vi "GetMotorHall.vi"(7 "Hall AI":dbl[][](array[numeric]), 8 "Hall状态输入":bool[](array[boolean]), 9 "电流输入":dbl[](array[numeric]), 11 "hall in":i64[](array[numeric])) -> (0 "Hall状态输出":bool[](array[boolean]), 1 "电流输出":dbl[](array[numeric]), 3 "Hall out":i64[](array[numeric]))   [LabVIEW 2018]
uses:
  <vilib>/Analysis/baseanly.llb/Mean (DBL).vi
  <vilib>/Analysis/NI_AALBase.lvlib
panel:
  out "ST55数组":dbl[][](array[numeric])
  out "ST45数组":dbl[][](array[numeric])
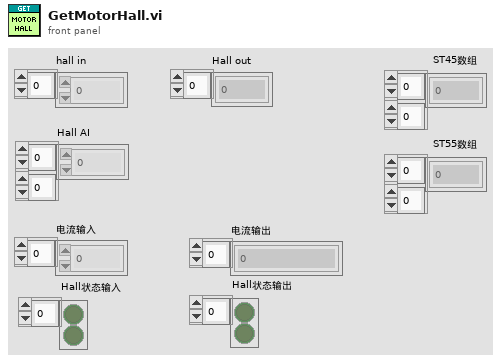
[diagram p1: front panel]
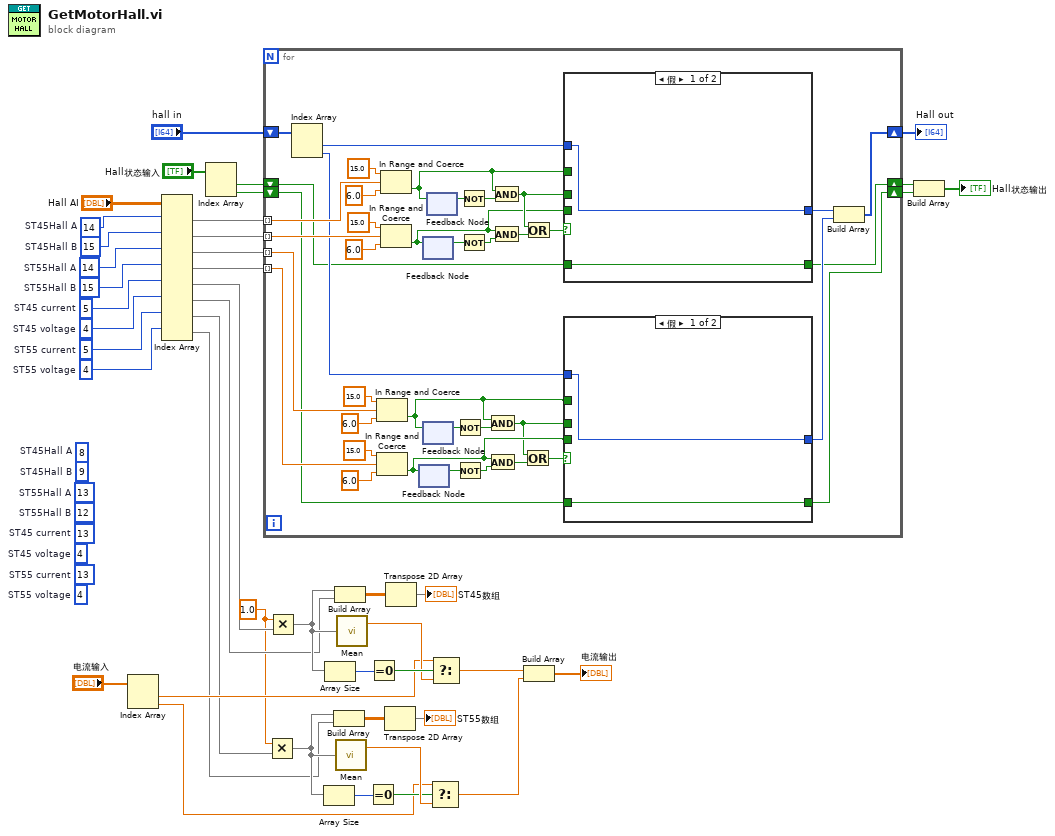
[diagram p0: block diagram]
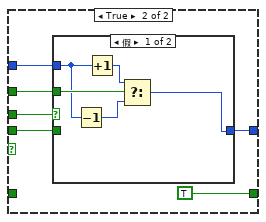
[diagram p2: hidden frame]
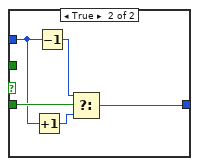
[diagram p3: hidden frame]
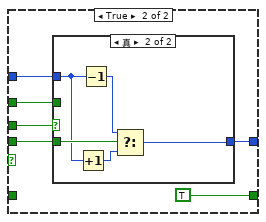
[diagram p4: hidden frame]
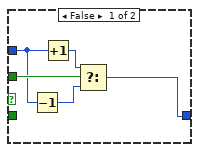
[diagram p5: hidden frame]
diagram:
  (unwired) 4  # ST55 voltage
  (unwired) 13  # ST55 current
  (unwired) 4  # ST45 voltage
  (unwired) 13  # ST45 current
  (unwired) 12  # ST55Hall B
  (unwired) 9  # ST45Hall B
  (unwired) 8  # ST45Hall A
  (unwired) 13  # ST55Hall A
  w26 = 4  # ST55 voltage
  w27 = 5  # ST55 current
  w10 = 1.0
  w28 = 4  # ST45 voltage
  w29 = 5  # ST45 current
  w30 = 15  # ST55Hall B
  w34 = 15  # ST45Hall B
  w35 = 14  # ST45Hall A
  w31 = 14  # ST55Hall A
  n1 = Index Array(array="电流输入") -> (element #1=w20:dbl, element #2=w8:dbl)  [unwired: 2 in]
  n2 = Index Array(array="Hall AI", index (row) #1=w35, index (row) #2=w34, index (row) #3=w31, index (row) #4=w30, index (row) #5=w29, index (row) #6=w28, index (row) #7=w27, index (row) #8=w26) -> (element #1=w38:dbl[], element #2=w37:dbl[], element #3=w23:dbl[], element #4=w22:dbl[], element #5=w24:dbl[], element #6=w25:dbl[], element #7=w11:dbl[], element #8=w9:dbl[])  [unwired: 8 in]
  n3 = Index Array(array="Hall状态输入") -> (element #1=w5:bool, element #2=w4:bool)  [unwired: 2 in]
  n4 = for {
    tunnel: w38 -> [w80] mode=indexing
    tunnel: w37 -> [w76] mode=indexing
    shift-right: [w65] -> w32
    shift-left: "hall in" -> [w70]
    tunnel: w23 -> [w52] mode=indexing
    tunnel: w22 -> [w51] mode=indexing
    shift-right: [w46] -> w3
    shift-left: w5 -> [w48]
    shift-right: [w45] -> w2
    shift-left: w4 -> [w47]
    n5 = Index Array(array=w70) -> (element #1=w69:i64, element #2=w68:i64)  [unwired: 2 in]
    n6 = In Range and Coerce(upper limit=15.0 ("上限"), x=w52, lower limit=6.0 ("下限")) -> (In Range?=w55:bool)  [unwired: 1 out]
    n7 = In Range and Coerce(upper limit=15.0 ("上限"), x=w51, lower limit=6.0 ("下限")) -> (In Range?=w54:bool)  [unwired: 1 out]
    n8 = In Range and Coerce(upper limit=15.0 ("上限"), x=w80, lower limit=6.0 ("下限")) -> (In Range?=w71:bool)  [unwired: 1 out]
    n9 = In Range and Coerce(upper limit=15.0 ("上限"), x=w76, lower limit=6.0 ("下限")) -> (In Range?=w72:bool)  [unwired: 1 out]
    n10 = feedback #1() -> (w62:bool)  [unwired: 1 in]
    n11 = feedback-in #1(w54) -> ()
    n12 = feedback #2() -> (w77:bool)  [unwired: 1 in]
    n13 = feedback-in #2(w72) -> ()
    n14 = feedback #3() -> (w57:bool)  [unwired: 1 in]
    n15 = feedback-in #3(w55) -> ()
    n16 = feedback #4() -> (w83:bool)  [unwired: 1 in]
    n17 = feedback-in #4(w71) -> ()
    n18 = Not(x=w57) -> (.not. x?=w56:bool)
    n19 = Not(x=w62) -> (.not. x?=w63:bool)
    n20 = Not(x=w83) -> (.not. x?=w84:bool)
    n21 = Not(x=w77) -> (.not. x?=w75:bool)
    n22 = And(x=w55, y=w56) -> (x .and. y?=w53:bool)
    n23 = And(x=w54, y=w63) -> (x .and. y?=w64:bool)
    n24 = And(x=w71, y=w84) -> (x .and. y?=w73:bool)
    n25 = And(x=w72, y=w75) -> (x .and. y?=w74:bool)
    n26 = Or(x=w53, y=w64) -> (x .or. y?=w49:bool)
    n27 = Or(x=w73, y=w74) -> (x .or. y?=w50:bool)
    n28 = case shown="假" w50 {
      tunnel: w69 -> [w104 w108]
      tunnel: w73 -> [_ w110]
      tunnel: w72 -> [_ w109]
      tunnel: [w104 w107] -> w67
      tunnel: w71 -> [_ w106]
      tunnel: [w103 TRUE] -> w46
      tunnel: w48 -> [w103 _]
      frame False {
      }
      frame True {
        n29 = case shown="真" w110 {
          tunnel: w109 -> [_ w120]
          tunnel: w108 -> [w112 w118]
          tunnel: [w114 w119] -> w107
          tunnel: w106 -> [w115 _]
          frame False {
            n30 = Decrement(x=w112) -> (x-1=w113:i64)
            n31 = Increment(x=w112) -> (x+1=w111:i64)
            n32 = Select(t=w111, s=w115, f=w113) -> (s? t:f=w114:i64)
          }
          frame True {
            n33 = Increment(x=w118) -> (x+1=w117:i64)
            n34 = Decrement(x=w118) -> (x-1=w116:i64)
            n35 = Select(t=w116, s=w120, f=w117) -> (s? t:f=w119:i64)
          }
        }
      }
    }
    n36 = case shown="假" w49 {
      tunnel: w68 -> [w86 w90]
      tunnel: w53 -> [_ w92]
      tunnel: w54 -> [_ w91]
      tunnel: [w86 w89] -> w66
      tunnel: w55 -> [_ w88]
      tunnel: w47 -> [w85 _]
      tunnel: [w85 TRUE] -> w45
      frame False {
      }
      frame True {
        n37 = case shown="假" w92 {
          tunnel: w91 -> [_ w102]
          tunnel: w90 -> [w94 w100]
          tunnel: [w96 w101] -> w89
          tunnel: w88 -> [w97 _]
          frame False {
            n38 = Decrement(x=w94) -> (x-1=w95:i64)
            n39 = Increment(x=w94) -> (x+1=w93:i64)
            n40 = Select(t=w93, s=w97, f=w95) -> (s? t:f=w96:i64)
          }
          frame True {
            n41 = Increment(x=w100) -> (x+1=w99:i64)
            n42 = Decrement(x=w100) -> (x-1=w98:i64)
            n43 = Select(t=w98, s=w102, f=w99) -> (s? t:f=w101:i64)
          }
        }
      }
    }
    n44 = Build Array(w67, w66) -> (w65:i64[])
  }
  "Hall out" <- w32
  n45 = Multiply(x=w10, y=w11) -> (x*y=w17:dbl[])
  n46 = Multiply(x=w10, y=w24) -> (x*y=w36:dbl[])
  n47 = Array Size(array=w17) -> (size(s)=w12:i32)
  n48 = Array Size(array=w36) -> (size(s)=w43:i32)
  n49 = Build Array(w17, w9) -> (w15:dbl[][])
  n50 = Build Array(w36, w25) -> (w40:dbl[][])
  n51 = call-poly <vilib>:"Mean.vi"("X"=w17) -> ("mean"=w14:dbl)  [unwired: 1 out]
  n52 = call-poly <vilib>:"Mean.vi"("X"=w36) -> ("mean"=w41:dbl)  [unwired: 1 out]
  n53 = Equal To 0?(x=w12) -> (x = 0?=w13:bool)
  n54 = Equal To 0?(x=w43) -> (x = 0?=w42:bool)
  n55 = Transpose 2D Array(2D array=w15) -> (transposed array=→"ST55数组":dbl[][])
  n56 = Transpose 2D Array(2D array=w40) -> (transposed array=→"ST45数组":dbl[][])
  n57 = Select(t=w8, s=w13, f=w14) -> (s? t:f=w7:dbl)
  n58 = Select(t=w20, s=w42, f=w41) -> (s? t:f=w19:dbl)
  n59 = Build Array(w19, w7) -> (→"电流输出":dbl[])
  n60 = Build Array(w3, w2) -> (→"Hall状态输出":bool[])
